vi "setPinDirYldrm.vi"(2 "YLDRMErrorInp":errorcluster, 3 "dir":u8, 4 "pin":u8, 5 "YLDRMPortInp":refnum<visa-resource-name>) -> (0 "YLDRMErrorOut":errorcluster, 1 "YLDRMPortOut":refnum<visa-resource-name>)   [LabVIEW 2015]
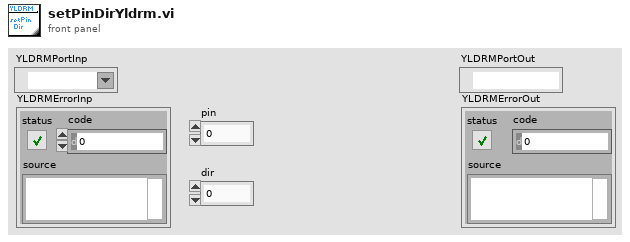
[diagram p1: front panel]
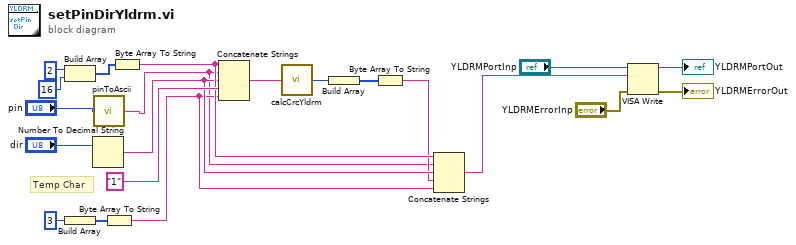
[diagram p0: block diagram]
diagram:
  # "Temp Char"
  n1 = Build Array(2, 16) -> (w19:i32[])
  n2 = Build Array(3) -> (w15:i32[])
  n3 = Number To Decimal String(number="dir") -> (decimal integer string=w6:string)  [unwired: 1 in]
  n4 = call "pinToAscii.vi"("inp"="pin") -> ("out"=w1:string)
  n5 = Byte Array To String(unsigned byte array=w15) -> (string=w4:string)
  n6 = Byte Array To String(unsigned byte array=w19) -> (string=w7:string)
  n7 = Concatenate Strings(w7, w1, w6, "1", w4) -> (w12:string)
  n8 = call "calcCrcYldrm.vi"("inpStr"=w12) -> ("crcVal"=w14:u8)
  n9 = Build Array(w14) -> (w13:u8[])
  n10 = Byte Array To String(unsigned byte array=w13) -> (string=w5:string)
  n11 = Concatenate Strings(w7, w1, w6, w5, w4) -> (w3:string)
  n12 = VISA Write(VISA resource name="YLDRMPortInp", write buffer=w3, error in (no error)="YLDRMErrorInp") -> (VISA resource name out=→"YLDRMPortOut":refnum<visa-resource-name>, error out=→"YLDRMErrorOut":errorcluster)  [unwired: 1 out]
